vi "Broadcast Panel State.vi"(8 "error in (no error)":errorcluster, 10 "Message":string, 11 "View In":refnum<class "View.lvclass">) -> (0 "error out":errorcluster, 3 "View Out":refnum<class "View.lvclass">)   [LabVIEW 2020, in "View.lvclass"]
uses:
  View.lvclass
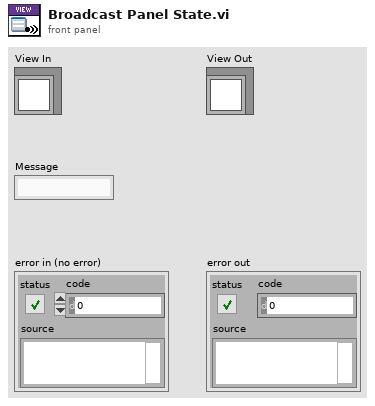
[diagram p1: front panel]
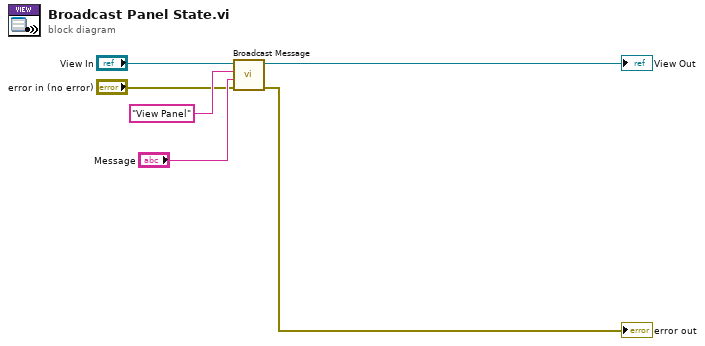
[diagram p0: block diagram]
diagram:
  n1 = call-dynamic "Broadcast Message.vi"("error in (no error)"="error in (no error)", "Message Data"="Message", "Message"="View Panel", "Process In"="View In") -> ("error out"=→"error out":errorcluster, "Process Out"=→"View Out":refnum<class "View.lvclass">)  [unwired: 6 in]
